vi "CVT Double IndexRead.vi"(3 "error in (no error)":errorcluster, 5 "Tag Index":i32) -> (0 "error out":errorcluster, 1 "Value":dbl)   [LabVIEW 2020, in "Current Value Table(Rebuild).lvlib"]
uses:
  Current Value Table(Rebuild).lvlib
  DataTypes/Double_Read Index.vi
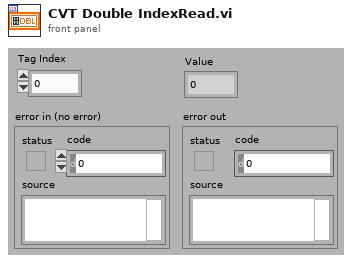
[diagram p1: front panel]
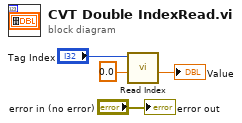
[diagram p0: block diagram]
diagram:
  n1 = call-poly "Read Index.vi"("Default"=0.0, "Index"="Tag Index") -> ("Value"=→"Value":dbl)  [unwired: 9 in]
  "error out" <- "error in (no error)"
